vi "T-F To OK-NG.vi"(11 "Result IN":bool) -> (3 "Result Out":string)   [LabVIEW 2021]
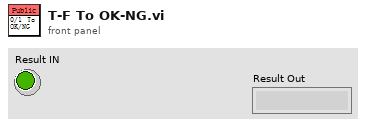
[diagram p1: front panel]
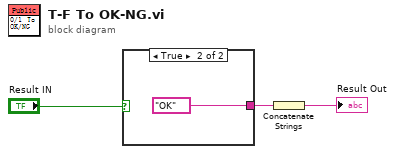
[diagram p0: block diagram]
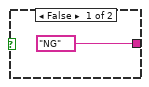
[diagram p2: hidden frame]
diagram:
  n1 = case shown="True" "Result IN" {
    tunnel: ["NG" ("Result") "OK" ("Result")] -> w3
    frame False {
    }
    frame True {
    }
  }
  n2 = Concatenate Strings(w3) -> (→"Result Out":string)
